vi "GV pretrigger clock.vi"() -> ()   [LabVIEW 2017]
panel:
  out "Pretrigger clock":bool
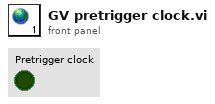
[diagram p1: front panel]
diagram:
